vi "Handle Error.vi"(8 "error in (no error)":errorcluster, 11 "TCP Stream in":refnum<class "TCP Stream.lvclass">) -> (0 "error out":errorcluster, 3 "TCP Stream out":refnum<class "TCP Stream.lvclass">)   [LabVIEW 2020, in "Stream-TCP.lvlib" / "TCP Stream.lvclass"]
uses:
  TCP Stream.lvclass
  Client Command.ctl
  TCP Stream.lvclass/TCP Stream.ctl
  Stream-TCP.lvlib
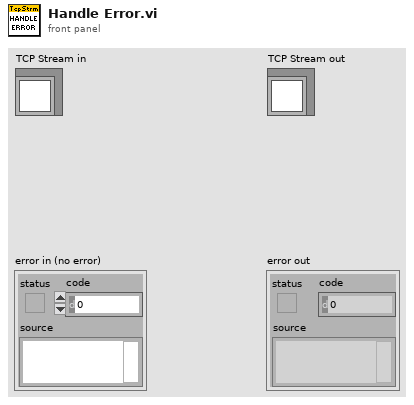
[diagram p1: front panel]
types:
  T1 = typedef "Stream-TCP.lvlib/Client Command.ctl" = enum16{"Connect", "Close", "Shutdown", "Reconnect"}
  T2 = typedef "Stream-TCP.lvlib/TCP Stream.lvclass/Ref Data.ctl" = cluster{"Client Command Queue":T3}
  T3 = typedef "Stream-TCP.lvlib/Client Command Queue.ctl" = refnum<queue>
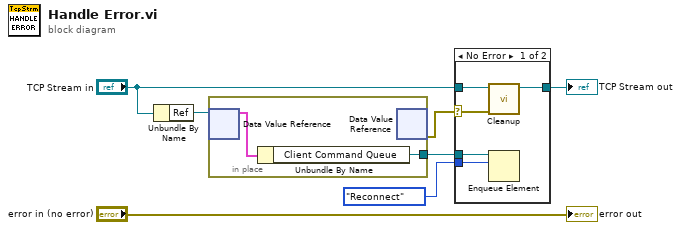
[diagram p0: block diagram]
diagram:
  n1 = Unbundle By Name("TCP Stream in") -> ("Ref"=w6:refnum<data-value>)
  n2 = in-place {
    in-place-border: [w8] -> w5
    n3 = in-place-dvr #1(w6) -> (w9:T2)  [unwired: 1 out]
    n4 = Unbundle By Name(w9) -> ("Client Command Queue"=w8:T3)
    n5 = in-place-dvr #1() -> (w1:errorcluster)  [unwired: 1 in, 1 out]
  }
  n6 = case shown="No Error" w1 {
    selector: w1 -> [w10 _]
    tunnel: w5 -> [w14 _]
    tunnel: Client_Command."Reconnect" ("element") -> [w13 _]
    tunnel: "TCP Stream in" -> [w12 w15]
    tunnel: [w11 w15] -> w2
    frame No Error {
      n7 = call-dynamic "Cleanup.vi"("error in (no error)"=w10, "TCP Stream in"=w12) -> ("TCP Stream out"=w11:refnum<class "TCP Stream.lvclass">)  [unwired: 8 in, 1 out]
      n8 = Enqueue Element(queue=w14, element=w13) -> ()  [unwired: 2 in, 3 out]
    }
    frame Error {
    }
  }
  "TCP Stream out" <- w2
  "error out" <- "error in (no error)"
